vi "SU_Get.vi"(6 "Direction":T1 items=["Positive", "Negative"], 8 "error in (no error)":errorcluster, 10 "Axis Number":i32, 11 "Agilis in":T2) -> (0 "error out":errorcluster, 2 "Step Amplitude":i32, 3 "Agilis out":T2)   [LabVIEW 2016, in "Drivers.lvlib" / "Agilis.lvlib"]
doc: "Sets the step amplitude (step size) in positive or negative direction."
uses:
  Agilis.lvlib
  AgilisCmdLib Refnum.ctl
  Direction.ctl
  Z:/TraceGrabber/Drivers/Agilis/AgilisCmdLib.dll
  AgilisCmdLib.dll
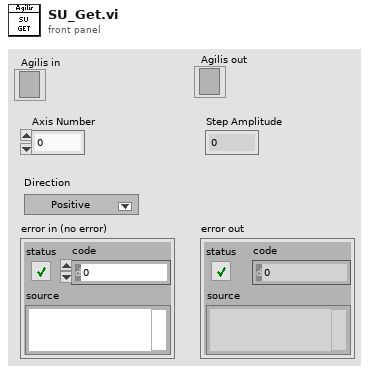
[diagram p1: front panel]
types:
  T1 = typedef "Drivers.lvlib/Agilis.lvlib/Direction.ctl" = u8
  T2 = typedef "Drivers.lvlib/Agilis.lvlib/AgilisCmdLib Refnum.ctl" = refnum<k24>
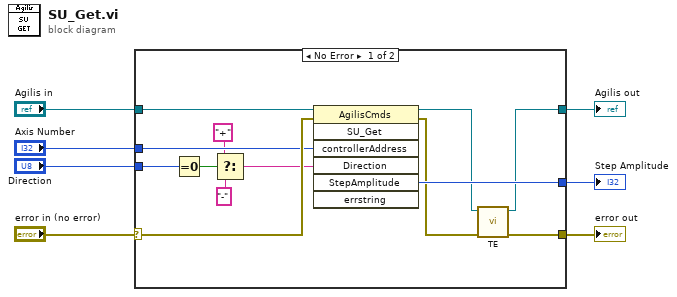
[diagram p0: block diagram]
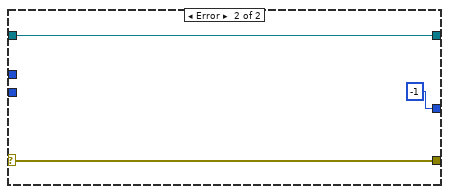
[diagram p2: hidden frame]
diagram:
  n1 = case shown="No Error" "error in (no error)" {
    selector: "error in (no error)" -> [w19 w23]
    tunnel: "Agilis in" -> [w20 w22]
    tunnel: [w8 w22] -> w5
    tunnel: [w10 w23] -> w4
    tunnel: "Axis Number" -> [w18 _]
    tunnel: [w17 -1 ("Target")] -> w2
    tunnel: "Direction" -> [w16 _]
    frame No Error {
      n2 = Equal To 0?(x=w16) -> (x = 0?=w15:bool)
      n3 = Select(t="+" ("Direction"), s=w15, f="-" ("Direction")) -> (s? t:f=w13:string)
      n4 = invoke class="AgilisCmds" method="SU_Get"(reference=w20, error in=w19, "controllerAddress"=w18, "Direction"=w13) -> (reference out=w9:T2, error out=w11:errorcluster, "StepAmplitude"=w17:i32)  [unwired: 3 in, 4 out]
      n5 = call "TE.vi"("error in (no error)"=w11, "Agilis in"=w9) -> ("error out"=w10:errorcluster, "Agilis out"=w8:T2)  [unwired: 8 in]
    }
    frame Error {
    }
  }
  "Agilis out" <- w5
  "error out" <- w4
  "Step Amplitude" <- w2
